vi "Feeder Oper.vi"   [LabVIEW 2016]
uses:
  Robot Global Data.vi
types:
  T1 = typedef "WPI_MotorControlDeviceRef.ctl" = cluster{"DeviceStatus":errorcluster, "Type":T2, "PWM":cluster{"PWM Channel":T3, "DeadBand":T4}, "CAN":cluster{"Device Number":u8, "SetOutput VI Ref":variant, "GetOutput VI Ref":variant, "Enable VI Ref":variant, "Disable VI Ref":variant, "Data":variant}, "Invert":bool}
  T2 = typedef "WPI_MotorControlType.ctl" = enum16{"PWM", "CAN"}
  T3 = typedef "FPGA_DIOPWMChannel.ctl" = enum8{"PWM 0", "PWM 1", "PWM 2", "PWM 3", "PWM 4", "PWM 5", "PWM 6", "PWM 7", "PWM 8", "PWM 9", "PWM MXP 0", "PWM MXP 1", "PWM MXP 2", "PWM MXP 3", "PWM MXP 4", "PWM MXP 5", "PWM MXP 6", "PWM MXP 7", "PWM MXP 8", "PWM MXP 9", "Invalid"}
  T4 = typedef "WPI_PWMDeadband.ctl" = cluster{"Name":string, "maxPositivePwm":i32, "minPositivePwm":i32, "centerPwm":i32, "maxNegativePwm":i32, "minNegativePwm":i32, "angularRange":u16}
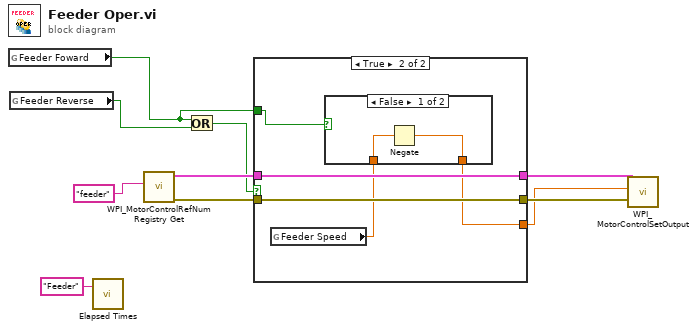
[diagram p0: block diagram]
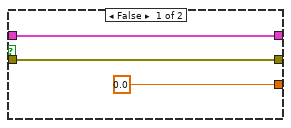
[diagram p2: hidden frame]
diagram:
  n1 = global read "Robot Global Data.vi" "Feeder Foward"() -> (w2:bool)
  n2 = global read "Robot Global Data.vi" "Feeder Reverse"() -> (w4:bool)
  n3 = call "Elapsed Times.vi"("Call Name"="Feeder") -> ()  [unwired: 2 in, 1 out]
  n4 = call <vilib>:"WPI_MotorControlRefNum Registry Get.vi"("refnum name"="feeder") -> ("error out"=w8:errorcluster, "MotorControlDevRef"=w9:T1)  [unwired: 9 in]
  n5 = Or(x=w2, y=w4) -> (x .or. y?=w3:bool)
  n6 = case shown="True" w3 {
    tunnel: w9 -> [w13 w18]
    tunnel: w8 -> [w12 w17]
    tunnel: [w13 w18] -> w7
    tunnel: [w12 w17] -> w6
    tunnel: [0.0 ("Output") w14] -> w5
    tunnel: w2 -> [_ w16]
    frame False {
    }
    frame True {
      n7 = global read "Robot Global Data.vi" "Feeder Speed"() -> (w15:dbl)
      n8 = case shown="False" w16 {
        tunnel: [w19 w21] -> w14
        tunnel: w15 -> [w20 w21]
        frame False {
          n9 = Negate(x=w20) -> (-x=w19:dbl)
        }
        frame True {
        }
      }
    }
  }
  n10 = call <vilib>:"WPI_MotorControlSetOutput.vi"("error in (no error)"=w6, "Output"=w5, "MotorControlDevRef"=w7) -> ()  [unwired: 6 in, 3 out]
